vi "ZMQ error augment.vi"(11 "error in":errorcluster) -> (3 "output cluster":errorcluster)   [LabVIEW 2018]
uses:
  <vilib>/addons/zeromq/zmq_libpath.vi
  <vilib>/Utility/error.llb/Error Cluster From Error Code.vi
  <vilib>/addons/zeromq/zeromq.lvlib
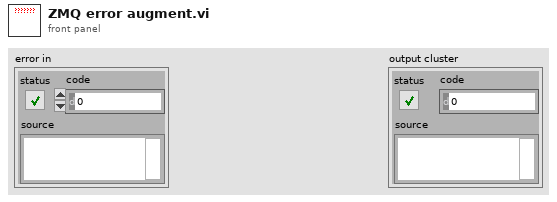
[diagram p1: front panel]
types:
  T1 = typedef "zeromq.lvlib/error_type.ctl" = enum16{"No Error", "EUNKNOWN", "ENOTSUP", "EPROTONOSUPPORT", "ENOBUFS", "ENETDOWN", "EADDRINUSE", "EADDRNOTAVAIL", "ECONNREFUSED", "EINPROGRESS", "ENOTSOCK", "EMSGSIZE", "EAFNOSUPPORT", "ENETUNREACH", "ECONNABORT", "ECONNRESET", "ENOTCONN", "ETIMEDOUT", "EHOSTUNREACH", "ENETRESET", "EBUSY", "EINVAL", "ENODEV", "EFAULT", "EINTR", "ENOENT", "ENOMEM", "EAGAIN", "EMFILE", "EFSM", "ENOCOMPATPROTO", "ETERM", "EMTHREAD", "Invalid"}
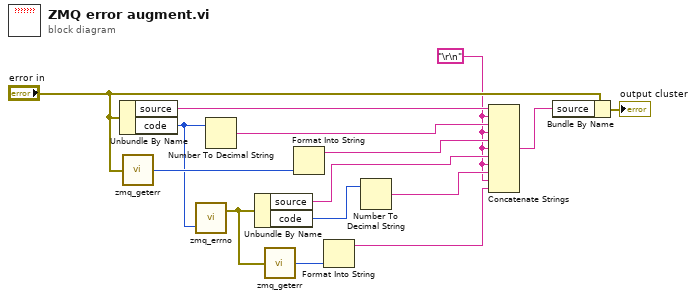
[diagram p0: block diagram]
diagram:
  w3 = "\r\n"
  n1 = Unbundle By Name("error in") -> ("source"=w11:string, "code"=w9:i32)
  n2 = call <vilib>:"zmq_geterr.vi"("error in"="error in") -> ("type"=w15:T1)
  n3 = call <vilib>:"zmq_errno.vi"("retval"=w9) -> ("error out"=w13:errorcluster)  [unwired: 1 in, 1 out]
  n4 = Number To Decimal String(number=w9) -> (decimal integer string=w8:string)  [unwired: 1 in]
  n5 = Unbundle By Name(w13) -> ("source"=w6:string, "code"=w5:i32)
  n6 = call <vilib>:"zmq_geterr.vi"("error in"=w13) -> ("type"=w12:T1)
  n7 = Format Into String(w15) -> (resulting string=w7:string)  [unwired: 3 in, 1 out]
  n8 = Format Into String(w12) -> (resulting string=w2:string)  [unwired: 3 in, 1 out]
  n9 = Number To Decimal String(number=w5) -> (decimal integer string=w4:string)  [unwired: 1 in]
  n10 = Concatenate Strings(w11, w3, w8, w3, w7, w3, w6, w3, w4, w3, w2) -> (w10:string)
  n11 = Bundle By Name(cluster="error in", "source"=w10) -> (→"output cluster":errorcluster)
